vi "Sensor color.vi"() -> ()   [LabVIEW 2017]
uses:
  enumColor.ctl
  <vilib>/DAQmx/write.llb/DAQmx Write (Digital 1D Bool 1Chan 1Samp).vi
  <vilib>/DAQmx/read.llb/DAQmx Read (Digital Bool 1Line 1Point).vi
  <vilib>/DAQmx/create/channels.llb/DAQmx Create Channel (DO-Digital Output).vi
  <vilib>/DAQmx/create/channels.llb/DAQmx Create Channel (DI-Digital Input).vi
  <vilib>/DAQmx/miscellaneous.llb/DAQmx Fill In Error Info.vi
panel:
  in  "Boolean":bool
  out "data":bool
  out "Azul":dbl
  out "Verde":dbl format="%.2f"
  out "Rojo":dbl format="%.2f"
  in  "Frecuencia 1":bool
  in  "Frecuencia 2":bool
  in  "stop":bool
  in  "Inicio":bool
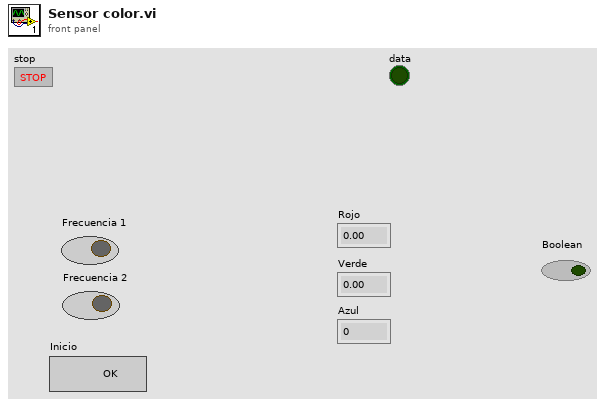
[diagram p1: front panel]
types:
  T1 = typedef "enumColor.ctl" = enum16{"Inicio", "Rojo1", "Rojo2", "Rojo3", "Verde1", "Verde2", "Verde3", "Azul1", "Azul2", "Azul3", "Cierre"}
  T2 = cluster{"task out":refnum<k21>, "error out":errorcluster}
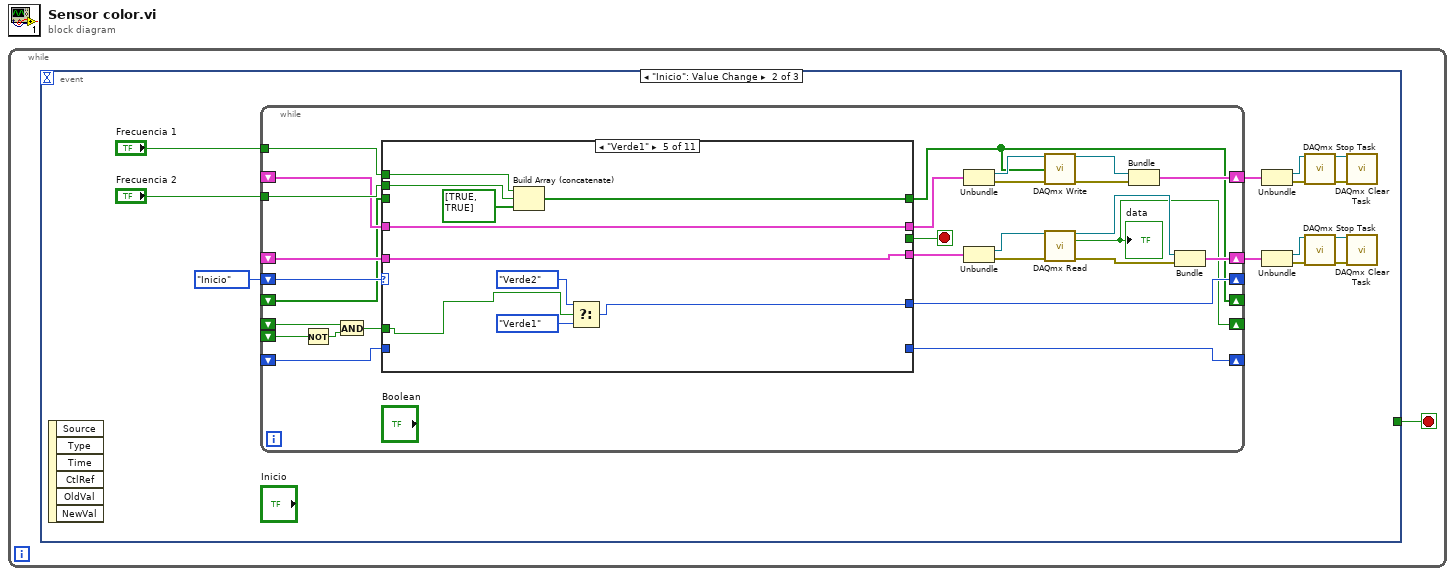
[diagram p0: block diagram]
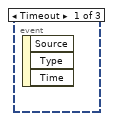
[diagram p2: hidden frame]
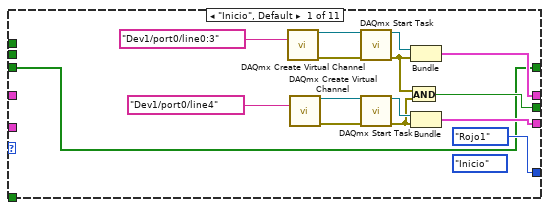
[diagram p3: hidden frame]
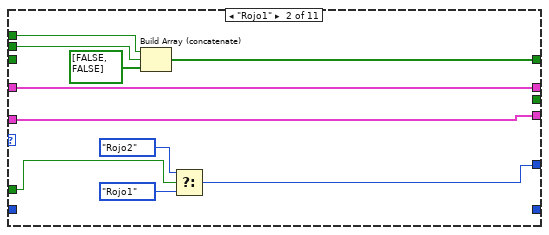
[diagram p4: hidden frame]
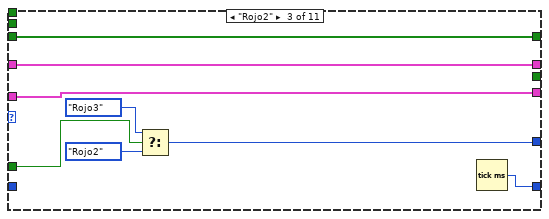
[diagram p5: hidden frame]
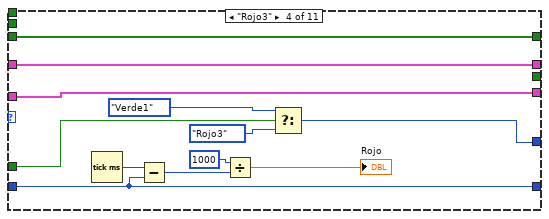
[diagram p6: hidden frame]
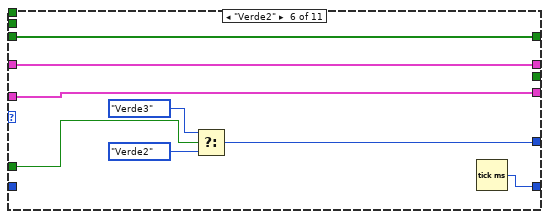
[diagram p7: hidden frame]
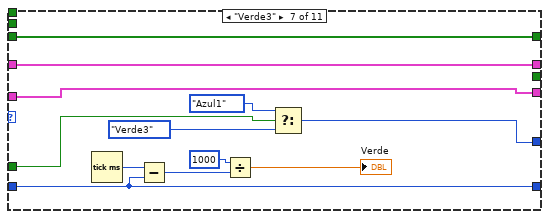
[diagram p8: hidden frame]
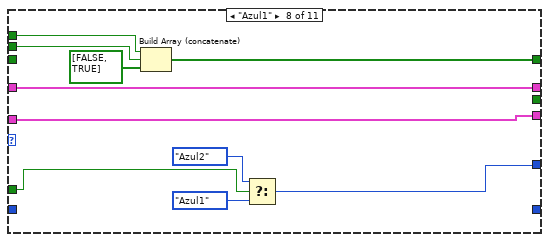
[diagram p9: hidden frame]
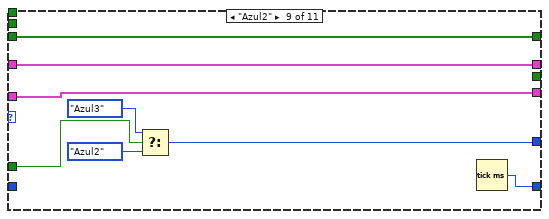
[diagram p10: hidden frame]
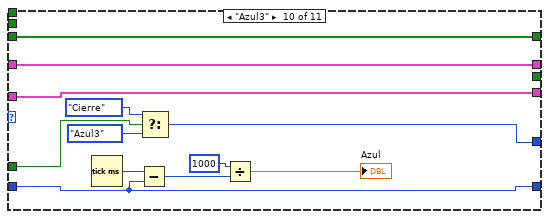
[diagram p11: hidden frame]
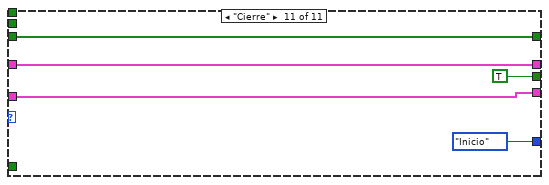
[diagram p12: hidden frame]
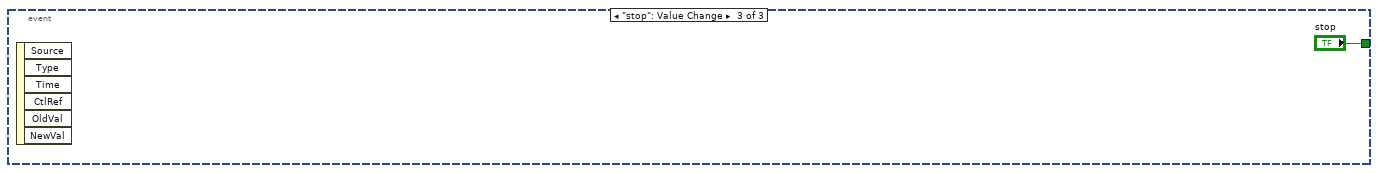
[diagram p13: hidden frame]
diagram:
  n1 = while {
    stop <- w1 stop-if-true
    n2 = event shown="[1] \"Inicio\": Value Change" {
      selector: _ -> [_ _ _]
      dyn-events: _ -> [_ _ _]
      timeout: _ -> [_ _ _]
      tunnel: [_ _ "stop"] -> w1
      event Timeout {
        n3 = event-data() -> ()  [unwired: 1 in, 3 out]
      }
      event "Inicio": Value Change {
        n4 = event-data() -> ()  [unwired: 1 in, 6 out]
        n5 = while {
          shift-right: [w41] -> _
          shift-left: enumColor."Inicio" -> [w20]
          shift-right: [w23] -> w12
          shift-left: _ -> [w26]
          shift-right: [w35] -> w11
          shift-left: _ -> [w30]
          tunnel: "Frecuencia 1" -> [w32]
          tunnel: "Frecuencia 2" -> [w31]
          shift-right: [w19] -> _
          shift-left: _ -> [w18]
          shift-left: _ -> [w17]
          shift-right: [w22] -> _
          shift-left: _ -> [w21]
          shift-right: [w16] -> _
          shift-left: _ -> [w15]
          stop <- w42 stop-if-true
          n6 = Not(x=w18) -> (.not. x?=w25:bool)
          n7 = And(x=w17, y=w25) -> (x .and. y?=w24:bool)
          n8 = case shown="\"Verde1\"" w20 {
            tunnel: [w53 _ _ _ _ _ _ _ _ _ TRUE] -> w42
            tunnel: [w46 w63 w75 w86 w92 w105 w111 w122 w135 w141 w151] -> w38
            tunnel: [enumColor."Rojo1" w58 w70 w81 w88 w99 w114 w118 w130 w146 enumColor."Inicio"] -> w41
            tunnel: w32 -> [_ w66 _ _ w96 _ _ w126 _ _ _]
            tunnel: w31 -> [_ w65 _ _ w95 _ _ w125 _ _ _]
            tunnel: [w43 w64 w68 w76 w94 w98 w106 w124 w128 w136 w148] -> w16
            tunnel: w30 -> [_ w63 w75 w86 w92 w105 w111 w122 w135 w141 w151]
            tunnel: [w44 w62 w74 w87 w93 w104 w112 w123 w134 w142 w152] -> w27
            tunnel: w26 -> [_ w62 w74 w87 w93 w104 w112 w123 w134 w142 w152]
            tunnel: w24 -> [_ w59 w71 w84 w89 w100 w117 w119 w129 w147 _]
            tunnel: w21 -> [_ _ _ w80 _ _ w110 _ _ w140 _]
            tunnel: [_ _ w69 w80 _ w101 w110 _ w131 w140 _] -> w22
            tunnel: w15 -> [w43 _ w68 w76 _ w98 w106 _ w128 w136 w148]
            frame "Inicio", Default {
              (unwired) enumColor."Inicio"
              n9 = call-poly <vilib>:"DAQmx Create Virtual Channel.vi"("lines"=tag "Dev1/port0/line0:3") -> ("task out"=w57:refnum<k21>, "error out"=w56:errorcluster)  [unwired: 13 in]
              n10 = call-poly <vilib>:"DAQmx Create Virtual Channel.vi"("lines"=tag "Dev1/port0/line4") -> ("task out"=w55:refnum<k21>, "error out"=w54:errorcluster)  [unwired: 13 in]
              n11 = call <vilib>:"DAQmx Start Task.vi"("task/channels in"=w57, "error in"=w56) -> ("task out"=w50:refnum<k21>, "error out"=w49:errorcluster)  [unwired: 12 in]
              n12 = call <vilib>:"DAQmx Start Task.vi"("task/channels in"=w55, "error in"=w54) -> ("task out"=w48:refnum<k21>, "error out"=w47:errorcluster)  [unwired: 12 in]
              n13 = And(x=w49, y=w47) -> (x .and. y?=w53:bool)
              n14 = Bundle("task out"=w50, "error out"=w49) -> (w44:T2)  [unwired: 1 in]
              n15 = Bundle("task out"=w48, "error out"=w47) -> (w46:T2)  [unwired: 1 in]
            }
            frame "Rojo1" {
              n16 = Build Array (concatenate)(w66, w65, bool[] [FALSE, FALSE]) -> (w64:bool[])
              n17 = Select(t=enumColor."Rojo2", s=w59, f=enumColor."Rojo1") -> (s? t:f=w58:T1)
            }
            frame "Rojo2" {
              n18 = Select(t=enumColor."Rojo3", s=w71, f=enumColor."Rojo2") -> (s? t:f=w70:T1)
              n19 = Tick Count (ms)() -> (millisecond timer value=w69:u32)
            }
            frame "Rojo3" {
              n20 = Tick Count (ms)() -> (millisecond timer value=w85:u32)
              n21 = Subtract(x=w85, y=w80) -> (x-y=w78:u32)
              n22 = Divide(x=u32 1000, y=w78) -> (x/y=→"Rojo":dbl)
              n23 = Select(t=enumColor."Verde1", s=w84, f=enumColor."Rojo3") -> (s? t:f=w81:T1)
            }
            frame "Verde1" {
              n24 = Build Array (concatenate)(w96, w95, bool[] [TRUE, TRUE]) -> (w94:bool[])
              n25 = Select(t=enumColor."Verde2", s=w89, f=enumColor."Verde1") -> (s? t:f=w88:T1)
            }
            frame "Verde2" {
              n26 = Select(t=enumColor."Verde3", s=w100, f=enumColor."Verde2") -> (s? t:f=w99:T1)
              n27 = Tick Count (ms)() -> (millisecond timer value=w101:u32)
            }
            frame "Verde3" {
              n28 = Tick Count (ms)() -> (millisecond timer value=w113:u32)
              n29 = Subtract(x=w113, y=w110) -> (x-y=w108:u32)
              n30 = Divide(x=u32 1000, y=w108) -> (x/y=→"Verde":dbl)
              n31 = Select(t=enumColor."Azul1", s=w117, f=enumColor."Verde3") -> (s? t:f=w114:T1)
            }
            frame "Azul1" {
              n32 = Build Array (concatenate)(w126, w125, bool[] [FALSE, TRUE]) -> (w124:bool[])
              n33 = Select(t=enumColor."Azul2", s=w119, f=enumColor."Azul1") -> (s? t:f=w118:T1)
            }
            frame "Azul2" {
              n34 = Select(t=enumColor."Azul3", s=w129, f=enumColor."Azul2") -> (s? t:f=w130:T1)
              n35 = Tick Count (ms)() -> (millisecond timer value=w131:u32)
            }
            frame "Azul3" {
              n36 = Tick Count (ms)() -> (millisecond timer value=w143:u32)
              n37 = Subtract(x=w143, y=w140) -> (x-y=w139:u32)
              n38 = Select(t=enumColor."Cierre", s=w147, f=enumColor."Azul3") -> (s? t:f=w146:T1)
              n39 = Divide(x=1000, y=w139) -> (x/y=→"Azul":dbl)
            }
            frame "Cierre" {
            }
          }
          n40 = Unbundle(w27) -> ("task out"=w40:refnum<k21>, "error out"=w39:errorcluster)
          n41 = Unbundle(w38) -> ("task out"=w37:refnum<k21>, "error out"=w36:errorcluster)
          n42 = call-poly <vilib>:"DAQmx Write.vi"("task/channels in"=w40, "data"=w16, "error in"=w39) -> ("task out"=w29:refnum<k21>, "error out"=w28:errorcluster)  [unwired: 10 in, 1 out]
          n43 = call-poly <vilib>:"DAQmx Read.vi"("task/channels in"=w37, "error in"=w36) -> ("task out"=w34:refnum<k21>, "data"=w19:bool, "error out"=w33:errorcluster)  [unwired: 11 in]
          "data" <- w19
          n44 = Bundle("task out"=w29, "error out"=w28) -> (w23:T2)  [unwired: 1 in]
          n45 = Bundle("task out"=w34, "error out"=w33) -> (w35:T2)  [unwired: 1 in]
        }
        n46 = Unbundle(w12) -> ("task out"=w10:refnum<k21>, "error out"=w9:errorcluster)
        n47 = Unbundle(w11) -> ("task out"=w8:refnum<k21>, "error out"=w7:errorcluster)
        n48 = call <vilib>:"DAQmx Stop Task.vi"("task/channels in"=w10, "error in"=w9) -> ("task out"=w6:refnum<k21>, "error out"=w5:errorcluster)  [unwired: 12 in]
        n49 = call <vilib>:"DAQmx Stop Task.vi"("task/channels in"=w8, "error in"=w7) -> ("task out"=w4:refnum<k21>, "error out"=w3:errorcluster)  [unwired: 12 in]
        n50 = call <vilib>:"DAQmx Clear Task.vi"("task in"=w6, "error in"=w5) -> ()  [unwired: 13 in, 1 out]
        n51 = call <vilib>:"DAQmx Clear Task.vi"("task in"=w4, "error in"=w3) -> ()  [unwired: 13 in, 1 out]
      }
      event "stop": Value Change {
        n52 = event-data() -> ()  [unwired: 1 in, 6 out]
      }
    }
  }
